vi "Pre Launch Init.vi"(11 "Camera in":refnum<class "Camera.lvclass">) -> (0 "error out":errorcluster, 3 "Camera out":refnum<class "Camera.lvclass">)   [LabVIEW 2021, in "Camera.lvlib" / "Camera.lvclass"]
doc: "(<B>Filename</B>: Actor Framework.lvlib:Actor.lvclass:Pre Launch Init.vi)\n\nDefines behavior that occurs after the Launch Nested Actor method is invoked but before the actor's Actor Core method begins running.\n\nBy default, this method does nothing. A descendant class may override it to define behavior."
uses:
  Camera.lvclass
  C:/Program Files (x86)/National Instruments/LabVIEW 2021/vi.lib/ActorFramework/Actor/Actor.lvclass
  Utilities/RWC_Actions.ctl
  <vilib>/ActorFramework/Actor/Actor.lvclass/Actor.ctl
  <vilib>/ActorFramework/Message Enqueuer/Message Enqueuer.lvclass/Message Enqueuer.ctl
  <vilib>/ActorFramework/Report Error Msg/Report Error Msg.lvclass/Report Error Msg.ctl
  Camera.lvclass/Camera.ctl
  <vilib>/ActorFramework/Message Enqueuer/Enqueue.vi
  <vilib>/ActorFramework/Message Enqueuer/Init from Existing Queue.vi
  <vilib>/ActorFramework/Report Error Msg/Report Error Msg.lvclass
  C:/Program Files (x86)/National Instruments/LabVIEW 2021/vi.lib/ActorFramework/Message/Message.lvclass
  <vilib>/ActorFramework/Message Priority Queue/Priority Enqueue.vi
  <vilib>/ActorFramework/Message Enqueuer/Message Enqueuer.lvclass
  <vilib>/ActorFramework/Actor/Actor.lvclass
panel:
  in  "Cam inner parameters":T1
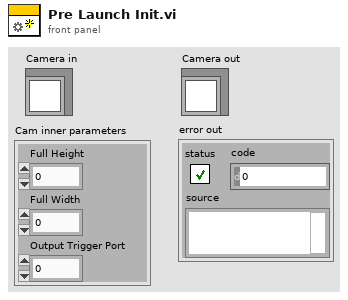
[diagram p1: front panel]
types:
  T1 = cluster{"Full Height":dbl, "Full Width":dbl, "Output Trigger Port":dbl}
  T2 = typedef "RWC_Actions.ctl" = enum16{"Read", "Write", "Read and Create"}
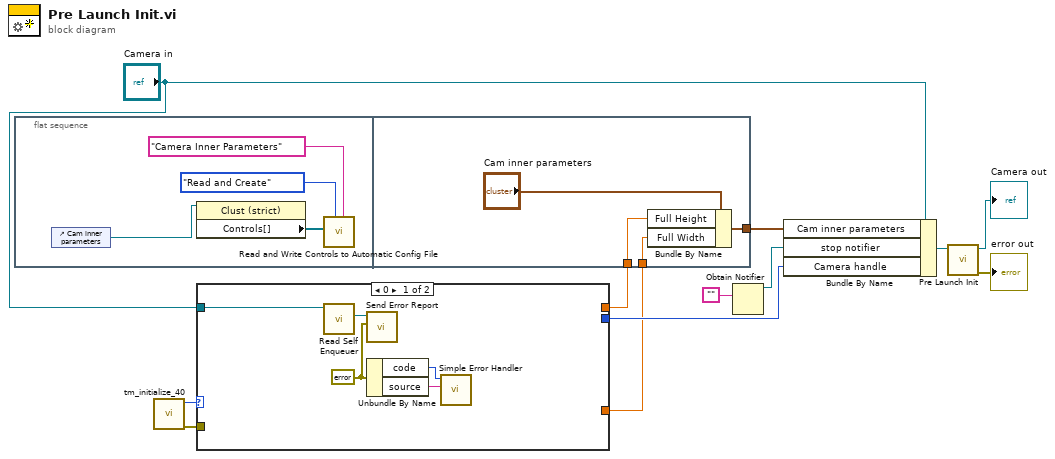
[diagram p0: block diagram]
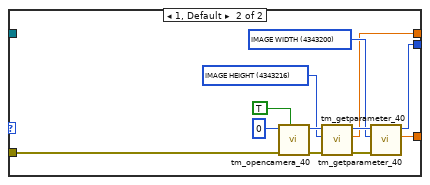
[diagram p2: hidden frame]
diagram:
  n1 = flat-sequence {
    tunnel: [w19] -> w3
    tunnel: w2 -> [w18]
    tunnel: w1 -> [w17]
    frame #0 {
      n2 = control-ref of="Cam inner parameters"() -> (w13:refnum<vi>)
      n3 = property class="Clust (strict)"(reference=w13) -> ("Controls[]"=w14:refnum<vi>[])  [unwired: 1 in, 2 out]
      n4 = call "Read and Write Controls to Automatic Config File.vi"("file name"="Camera Inner Parameters" ("section (optional)"), "Action"=RWC_Actions."Read and Create", "Control References"=w14) -> ()  [unwired: 8 in, 1 out]
    }
    frame #1 {
      n5 = Bundle By Name(cluster="Cam inner parameters", "Full Height"=w18, "Full Width"=w17) -> (w19:T1)
    }
  }
  n6 = call <userlib>:"tm_initialize_40.vi"() -> ("error out"=w7:errorcluster, "Number Of Cameras"=w6:u32)  [unwired: 8 in, 2 out]
  n7 = case shown="0" w6 {
    tunnel: w7 -> [_ w37]
    tunnel: "Camera in" -> [w24 _]
    tunnel: [_ w31] -> w5
    tunnel: [_ w27] -> w2
    tunnel: [_ w26] -> w1
    frame 0 {
      w23 = errorcluster {"status"=TRUE, "code"=8888, "source"="tm_initialize did not detect any connected camera"} ("Error From Sender")
      n8 = call <vilib>:"Read Self Enqueuer.vi"("Actor"=w24) -> ("Self Enqueuer"=w25:refnum<class "Message Enqueuer.lvclass">)  [unwired: 10 in]
      n9 = call <vilib>:"Send Error Report.vi"("Error From Sender"=w23, "Message Enqueuer"=w25) -> ()  [unwired: 9 in, 1 out]
      n10 = Unbundle By Name(w23) -> ("code"=w22:i32, "source"=w21:string)
      n11 = call <vilib>:"Simple Error Handler.vi"("error code (no error:0)"=w22, "error source (\" \")"=w21) -> ()  [unwired: 3 in, 5 out]
    }
    frame 1, Default {
      w28 = u32 4343200 items=["SENSOR MODE"=4212128, "READOUT SPEED"=4211872, "READOUT DIRECTION"=4211904, "TRIGGER GLOBAL EXPOSURE"=2049680, "TRIGGER DELAY"=1066480, "INTERNAL TRIGGER HANDLING"=1066496, "SENSOR TEMPERATURE"=2115232, "SENSOR COOLER STATUS"=2115280, "EXPOSURE TIME"=2049184, "DEFECT CORRECT MODE"=4670368, "HOT PIXEL CORRECT LEVEL"=4670400, "BINNING"=4215968, "TIMING READOUT TIME"=4223904, "INTERNAL FRAME RATE"=4225952, "INTERNAL FRAME INTERVAL"=4225968, "INTERNAL LINE SPEED"=4226000, "INTERNAL LINE INTERVAL"=4226016, "IMAGE WIDTH"=4343200, "IMAGE HEIGHT"=4343216, "IMAGE ROWBYTES"=4343232, "IMAGE FRAMEBYTES"=4343248, "IMAGE PIXEL TYPE"=4343296, "NUMBER OF OUTPUT TRIGGER CONNECTOR"=1852320, "OUTPUT TRIGGER SOURCE[0]"=1852576, "OUTPUT TRIGGER SOURCE[1]"=1852832, "OUTPUT TRIGGER SOURCE[2]"=1853088, "OUTPUT TRIGGER POLARITY[0]"=1852592, "OUTPUT TRIGGER POLARITY[1]"=1852848, "OUTPUT TRIGGER POLARITY[2]"=1853104, "OUTPUT TRIGGER ACTIVE[0]"=1852608, "OUTPUT TRIGGER ACTIVE[1]"=1852864, "OUTPUT TRIGGER ACTIVE[2]"=1853120, "OUTPUT TRIGGER DELAY[0]"=1852624, "OUTPUT TRIGGER DELAY[1]"=1852880, "OUTPUT TRIGGER DELAY[2]"=1853136, "OUTPUT TRIGGER PERIOD[0]"=1852640, "OUTPUT TRIGGER PERIOD[1]"=1852896, "OUTPUT TRIGGER PERIOD[2]"=1853152, "OUTPUT TRIGGER KIND[0]"=1852656, "OUTPUT TRIGGER KIND[1]"=1852912, "OUTPUT TRIGGER KIND[2]"=1853168, "OUTPUT TRIGGER BASE SENSOR[0]"=1852672, "OUTPUT TRIGGER BASE SENSOR[1]"=1852928, "OUTPUT TRIGGER BASE SENSOR[2]"=1853184, "OUTPUT TRIGGER PRE HSYNC COUNT"=1852704] ("Parameter")
      w29 = u32 4343216 items=["SENSOR MODE"=4212128, "READOUT SPEED"=4211872, "READOUT DIRECTION"=4211904, "TRIGGER GLOBAL EXPOSURE"=2049680, "TRIGGER DELAY"=1066480, "INTERNAL TRIGGER HANDLING"=1066496, "SENSOR TEMPERATURE"=2115232, "SENSOR COOLER STATUS"=2115280, "EXPOSURE TIME"=2049184, "DEFECT CORRECT MODE"=4670368, "HOT PIXEL CORRECT LEVEL"=4670400, "BINNING"=4215968, "TIMING READOUT TIME"=4223904, "INTERNAL FRAME RATE"=4225952, "INTERNAL FRAME INTERVAL"=4225968, "INTERNAL LINE SPEED"=4226000, "INTERNAL LINE INTERVAL"=4226016, "IMAGE WIDTH"=4343200, "IMAGE HEIGHT"=4343216, "IMAGE ROWBYTES"=4343232, "IMAGE FRAMEBYTES"=4343248, "IMAGE PIXEL TYPE"=4343296, "NUMBER OF OUTPUT TRIGGER CONNECTOR"=1852320, "OUTPUT TRIGGER SOURCE[0]"=1852576, "OUTPUT TRIGGER SOURCE[1]"=1852832, "OUTPUT TRIGGER SOURCE[2]"=1853088, "OUTPUT TRIGGER POLARITY[0]"=1852592, "OUTPUT TRIGGER POLARITY[1]"=1852848, "OUTPUT TRIGGER POLARITY[2]"=1853104, "OUTPUT TRIGGER ACTIVE[0]"=1852608, "OUTPUT TRIGGER ACTIVE[1]"=1852864, "OUTPUT TRIGGER ACTIVE[2]"=1853120, "OUTPUT TRIGGER DELAY[0]"=1852624, "OUTPUT TRIGGER DELAY[1]"=1852880, "OUTPUT TRIGGER DELAY[2]"=1853136, "OUTPUT TRIGGER PERIOD[0]"=1852640, "OUTPUT TRIGGER PERIOD[1]"=1852896, "OUTPUT TRIGGER PERIOD[2]"=1853152, "OUTPUT TRIGGER KIND[0]"=1852656, "OUTPUT TRIGGER KIND[1]"=1852912, "OUTPUT TRIGGER KIND[2]"=1853168, "OUTPUT TRIGGER BASE SENSOR[0]"=1852672, "OUTPUT TRIGGER BASE SENSOR[1]"=1852928, "OUTPUT TRIGGER BASE SENSOR[2]"=1853184, "OUTPUT TRIGGER PRE HSYNC COUNT"=1852704] ("Parameter")
      n12 = call <userlib>:"tm_opencamera_40.vi"("Force Open"=TRUE, "error in (no error)"=w37, "Camera Index"=u32 0) -> ("error out"=w30:errorcluster, "Handle out"=w34:u32)  [unwired: 6 in, 1 out]
      n13 = call <userlib>:"tm_getparameter_40.vi"("error in (no error)"=w30, "Parameter"=w29, "Handle in"=w34) -> ("error out"=w33:errorcluster, "Value out"=w27:dbl, "Handle out"=w32:u32)  [unwired: 6 in]
      n14 = call <userlib>:"tm_getparameter_40.vi"("error in (no error)"=w33, "Parameter"=w28, "Handle in"=w32) -> ("Value out"=w26:dbl, "Handle out"=w31:u32)  [unwired: 6 in, 1 out]
    }
  }
  n15 = Obtain Notifier(notification data type="") -> (notifier out=w9:refnum<notifier>)  [unwired: 3 in, 2 out]
  n16 = Bundle By Name(cluster="Camera in", "Cam inner parameters"=w3, "stop notifier"=w9, "Camera handle"=w5) -> (w8:refnum<class "Camera.lvclass">)
  n17 = call-parent "Pre Launch Init.vi"("Actor in"=w8) -> ("error out"=→"error out":errorcluster, "Actor out"=→"Camera out":refnum<class "Camera.lvclass">)  [unwired: 9 in]
